vi "Pack for gRPC.vi"(8 "error in":errorcluster, 9 "configuration / results":enum16{"Configuration", "Results"}(ring), 10 "data value":variant, 11 "measurement customizations in":refnum<class "Measurement Plugin.lvclass">) -> (0 "error out":errorcluster, 2 "any":T1, 3 "measurement customizations out":refnum<class "Measurement Plugin.lvclass">)   [LabVIEW 2021, in "Single Point_Channel Ganging.lvlib" / "Measurement Plugin.lvclass"]
uses:
  Measurement Plugin.lvclass
  Measurement Plugin.lvclass/Measurement Plugin.ctl
  Measurement Configuration.ctl
  Single Point_Channel Ganging.lvlib
  Measurement Results.ctl
  a6012965-5700-4384-8228-972e71b6560c.vi
  2eca732d-dbaa-43bf-a7dd-ede2da65bc1b.vi
  <vilib>/Plug-In SDKs/Measurements/Measurement Plugin Service/Measurement Plugin Service.lvclass
  C:/Program Files/National Instruments/LabVIEW 2021/vi.lib/Plug-In SDKs/Measurements/Measurement Plugin Service/Measurement Plugin Service.lvclass
  C:/Users/ngoli/Documents/pmic-labview/source/channel ganging/single point channel ganging/Single Point_Channel Ganging/Advanced/Measurement Plugin.lvclass
  <vilib>/gRPC/LabVIEW gRPC Library/Shared/Any.ctl
  <vilib>/gRPC/LabVIEW gRPC Library/grpc-lvsupport-release.lvlib
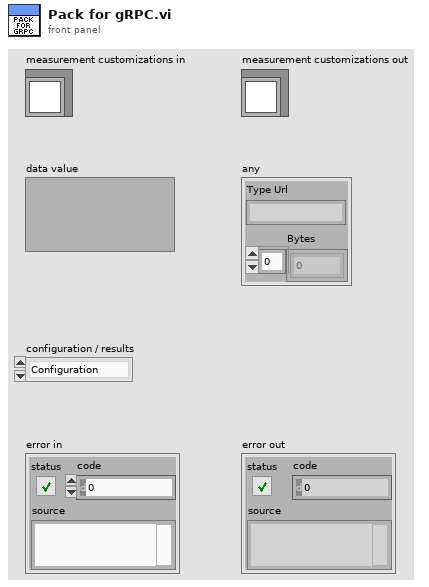
[diagram p1: front panel]
types:
  T1 = typedef "grpc-lvsupport-release.lvlib/Any.ctl" = cluster{"Type Url":string, "Bytes":u8[]}
  T2 = typedef "grpc-lvsupport-release.lvlib/grpcId.ctl" = u64
  T3 = typedef "Single Point_Channel Ganging.lvlib/Measurement Configuration.ctl" = cluster{"Source enable/disable":bool, "Load enable/disable":bool, "Source master resource name":string, "Source slave resource names":string[], "Load master resource name":string, "Load slave resource names":string[], "Source system configuration":enum32{"Series", "Parallel", "Manual"}, "Source output function":i32, "Source voltage/current level":dbl, "Source voltage/current level range":dbl, "Source sense":i32, "Source limit symmetry":enum32{"Symmetric", "Asymmetric"}, "Source current/voltage limit range":dbl, "Source current/voltage limit low":dbl, "Source current/voltage limit high":dbl, "Source transient response":i32, "Source voltage gain bandwidth":dbl, "Source voltage compensation frequency":dbl, "Source voltage pole-zero ratio":dbl, "Source current gain bandwidth":dbl, "Source current compensation frequency":dbl, "Source current pole-zero ratio":dbl, "Load system configuration":enum32{"Series", "Parallel", "Manual"}, "Load output function":i32, "Load voltage/current level":dbl, "Load voltage/current level range":dbl, "Load sense":i32, "Load limit symmetry":enum32{"Symmetric", "Asymmetric"}, "Load current/voltage limit range":dbl, "Load current/voltage limit low":dbl, "Load current/voltage limit high":dbl, "Load transient response":i32, "Load voltage gain bandwidth":dbl, "Load voltage compensation frequency":dbl, "Load voltage pole-zero ratio":dbl, "Load current gain bandwidth":dbl, "Load current compensation frequency":dbl, "Load current pole-zero ratio":dbl, "Load source trigger":string, "Aperture time":dbl, "Measurement time":dbl}
  T4 = typedef "Single Point_Channel Ganging.lvlib/Measurement Results.ctl" = cluster{"dt":dbl[], "Source voltages":dbl[], "Source currents":dbl[], "Load voltages":dbl[], "Load currents":dbl[], "Ganged source voltages":dbl[], "Ganged source currents":dbl[], "Ganged load voltages":dbl[], "Ganged load currents":dbl[], "Mean values":dbl[], "Minimum values":dbl[], "Maximum values":dbl[]}
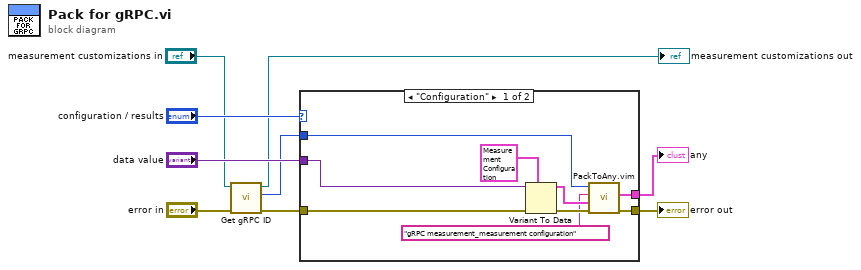
[diagram p0: block diagram]
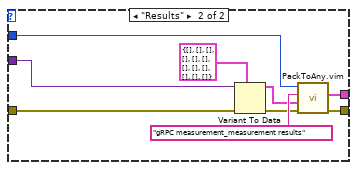
[diagram p2: hidden frame]
diagram:
  n1 = call <vilib>:"Get gRPC ID.vi"("error in"="error in", "measurement plugin service in"="measurement customizations in") -> ("error out"=w4:errorcluster, "gRPC ID"=w1:T2, "measurement plugin service out"=→"measurement customizations out":refnum<class "Measurement Plugin.lvclass">)  [unwired: 7 in]
  n2 = case shown="\"Configuration\"" "configuration / results" {
    tunnel: w4 -> [w18 w27]
    tunnel: "data value" -> [w17 w26]
    tunnel: w1 -> [w14 w22]
    tunnel: [w16 w24] -> w8
    tunnel: [w15 w23] -> w7
    frame "Configuration" {
      n3 = Variant To Data(error in=w18, type=T3 {"Source enable/disable"=TRUE, "Load enable/disable"=TRUE, "Source master resource name"="", "Source slave resource names"=[], "Load master resource name"="", "Load slave resource names"=[], "Source system configuration"=enum."Parallel", "Source output function"=2, "Source voltage/current level"=20.0, "Source voltage/current level range"=2.0, "Source sense"=0, "Source limit symmetry"=enum."Asymmetric", "Source current/voltage limit range"=2.0, "Source current/voltage limit low"=20.0, "Source current/voltage limit high"=2.0, "Source transient response"=2, "Source voltage gain bandwidth"=2000.0, "Source voltage compensation frequency"=3530.0, "Source voltage pole-zero ratio"=2.0, "Source current gain bandwidth"=20000.0, "Source current compensation frequency"=4000.0, "Source current pole-zero ratio"=1.0, "Load system configuration"=enum."Parallel", "Load output function"=20, "Load voltage/current level"=2.0, "Load voltage/current level range"=2.0, "Load sense"=0, "Load limit symmetry"=enum."Asymmetric", "Load current/voltage limit range"=20.0, "Load current/voltage limit low"=0.0, "Load current/voltage limit high"=inf, "Load transient response"=2, "Load voltage gain bandwidth"=10000.0, "Load voltage compensation frequency"=50000.0, "Load voltage pole-zero ratio"=12.0, "Load current gain bandwidth"=14000.0, "Load current compensation frequency"=180000.0, "Load current pole-zero ratio"=0.3, "Load source trigger"="", "Aperture time"=0.01, "Measurement time"=0.01} ("measurement configuration"), Variant=w17) -> (data=w13:T3, error out=w12:errorcluster)
      n4 = call "PackToAny.vim"("error in"=w12, "Data To Pack"=w13, "Message Type"="gRPC measurement_measurement configuration", "gRPCid in"=w14) -> ("error out"=w16:errorcluster, "Any"=w15:T1)  [unwired: 5 in, 1 out]
    }
    frame "Results" {
      n5 = Variant To Data(error in=w27, type=T4 {"dt"=[], "Source voltages"=[], "Source currents"=[], "Load voltages"=[], "Load currents"=[], "Ganged source voltages"=[], "Ganged source currents"=[], "Ganged load voltages"=[], "Ganged load currents"=[], "Mean values"=[], "Minimum values"=[], "Maximum values"=[]} ("Measurement Results"), Variant=w26) -> (data=w20:T4, error out=w19:errorcluster)
      n6 = call "PackToAny.vim"("error in"=w19, "Data To Pack"=w20, "Message Type"="gRPC measurement_measurement results", "gRPCid in"=w22) -> ("error out"=w24:errorcluster, "Any"=w23:T1)  [unwired: 5 in, 1 out]
    }
  }
  "error out" <- w8
  "any" <- w7
